vi "test_gs_v2.vi"() -> ()   [LabVIEW 2015]
uses:
  <vilib>/Native 3D Graph/xcontrol/3DPC_SurfacePlot.xctl
  <vilib>/Instr/_visa.llb/VISA Flush IO Buffer Mask.ctl
panel:
  in  "Tab Control":enum32{"Page 1", "Page 2"}(tab)
  in  "stop":bool
  out "x":string
  out "3D Graph":refnum<class "Base Datatype.lvclass">[](xcontrol)
  in  "Ramp Z to:":string(combo)
  in  "Ramp Y to:":string(combo)
  in  "Ramp X to:":string(combo)
  in  "Z-axis Persistence heater ON/OFF":bool
  in  "Y-axis Persistence heater ON/OFF":bool
  in  "Z-axis port name":refnum<visa-resource-name>
  in  "Y-axis port name":refnum<visa-resource-name>
  in  "X-axis Persistence heater ON/OFF":bool
  in  "X-axis port name":refnum<visa-resource-name>
  out "B_x":dbl
  out "B_y":dbl
  out "B_z":dbl
  in  "Field strength in Tesla":dbl min=0.0 max=9.0
  in  "beta in degrees 0 to   180":dbl min=0.0 max=180.0
  in  "alpha in degrees 0 to 360":dbl min=0.0 max=360.0
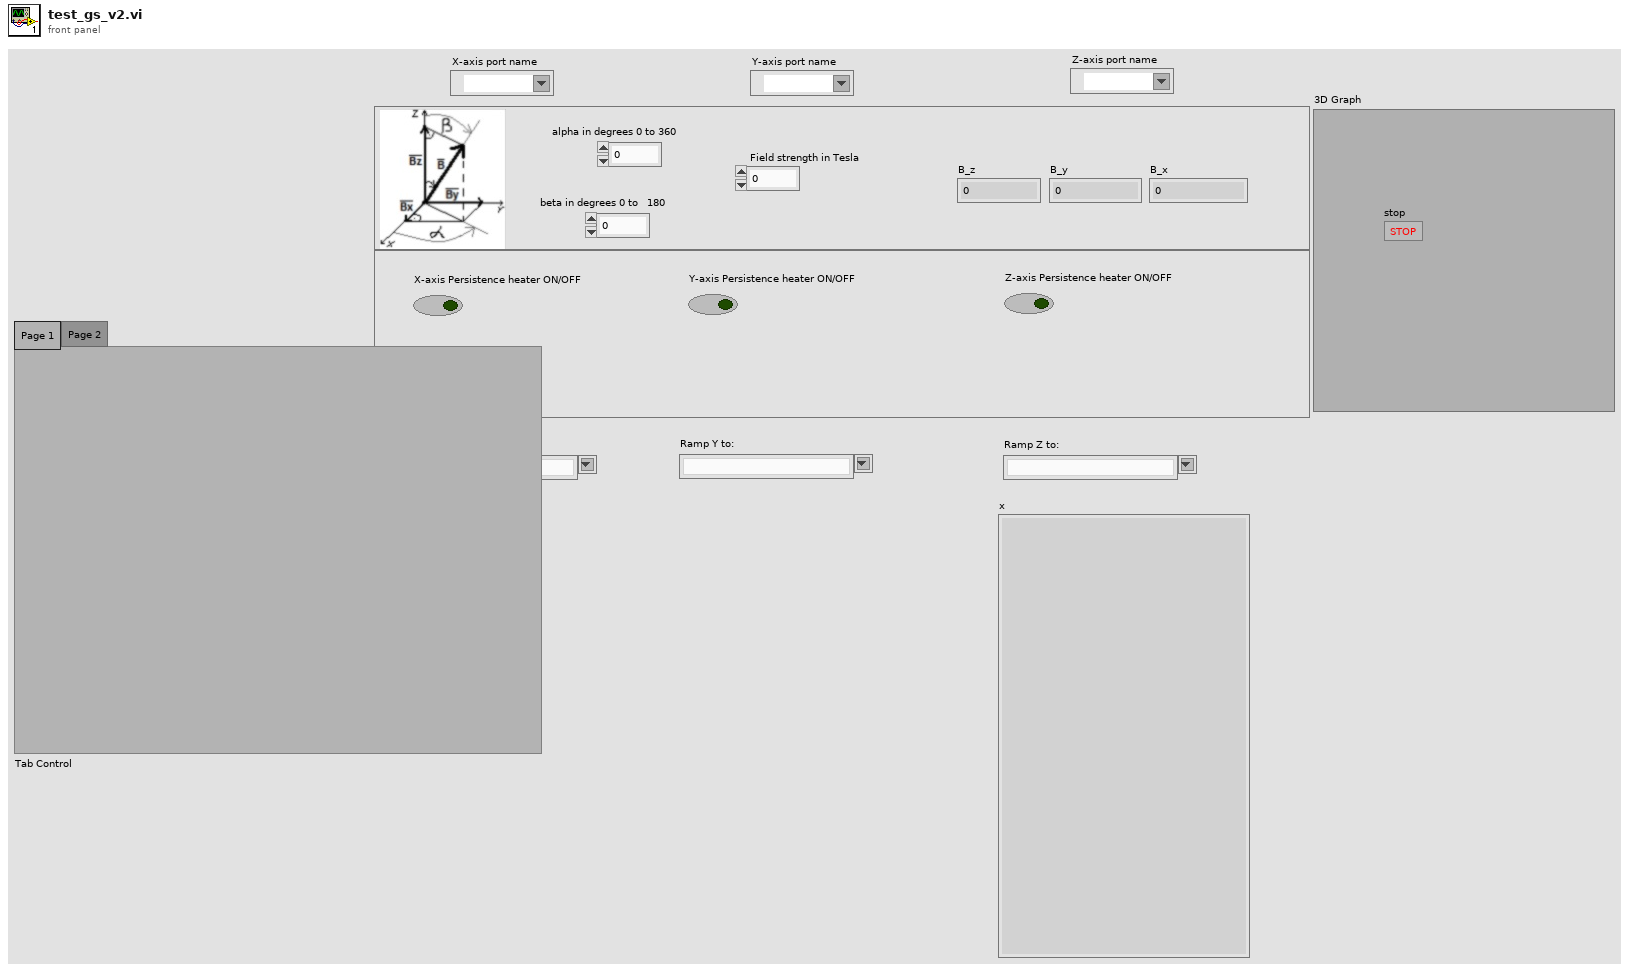
[diagram p1: front panel]
types:
  T1 = typedef "VISA Flush IO Buffer Mask.ctl" = u16
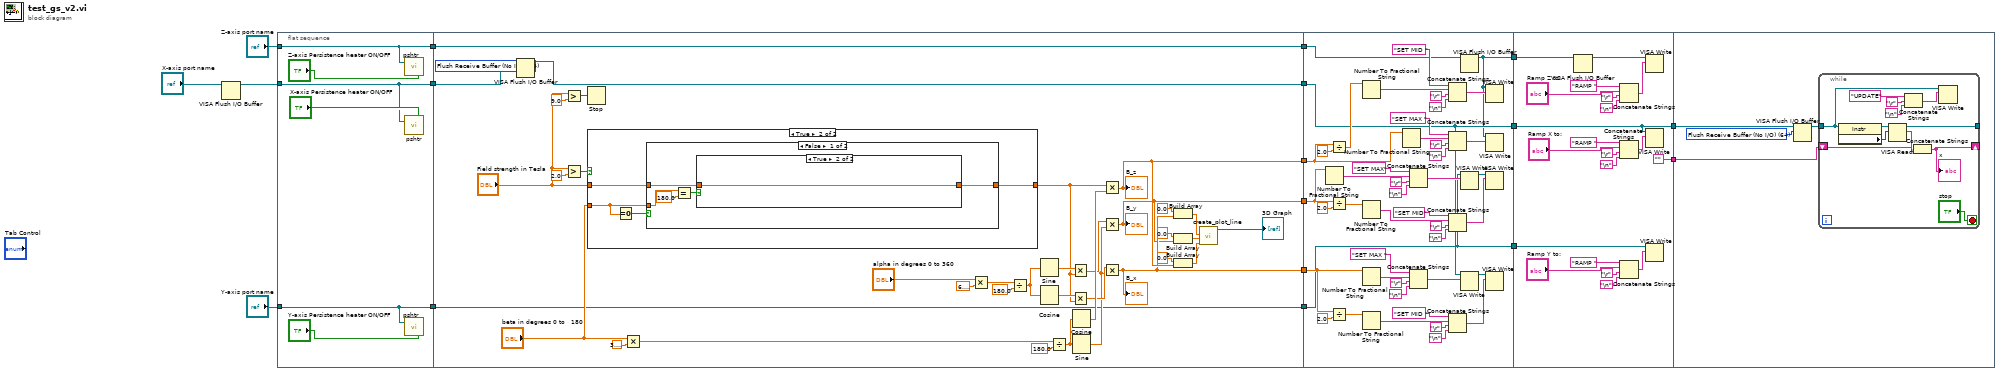
[diagram p0: block diagram]
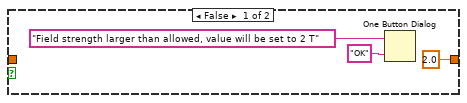
[diagram p3: hidden frame]
diagram:
  n1 = VISA Flush I/O Buffer(VISA resource name="X-axis port name") -> (VISA resource name out=w1:refnum<visa-resource-name>)  [unwired: 2 in, 1 out]
  n2 = flat-sequence {
    tunnel: "Z-axis port name" -> [w19]
    tunnel: "Y-axis port name" -> [w20]
    tunnel: w1 -> [w21]
    tunnel: [w21] -> w10
    tunnel: [w20] -> w9
    tunnel: [w19] -> w8
    tunnel: [w26] -> w16
    tunnel: [w33] -> w15
    tunnel: [w32] -> w14
    tunnel: [w31] -> w13
    tunnel: [w30] -> w12
    tunnel: [w29] -> w11
    tunnel: w10 -> [w27]
    tunnel: w9 -> [w33]
    tunnel: w8 -> [w32]
    tunnel: w16 -> [w84]
    tunnel: w15 -> [w83]
    tunnel: w14 -> [w78]
    tunnel: w13 -> [w89]
    tunnel: w12 -> [w91]
    tunnel: w11 -> [w88]
    tunnel: [w84] -> w7
    tunnel: [w83] -> w6
    tunnel: [w77] -> w5
    tunnel: w7 -> [w122]
    tunnel: w6 -> [w129]
    tunnel: w5 -> [w124]
    tunnel: [""] -> w4
    tunnel: [w122] -> w3
    tunnel: w4 -> [w145]
    tunnel: w3 -> [w144]
    frame #0 {
      n3 = call "pshtr.vi"("Boolean"="Z-axis Persistence heater ON/OFF", "VISA resource name"=w19) -> ()  [unwired: 1 in]
      n4 = call "pshtr.vi"("Boolean"="X-axis Persistence heater ON/OFF", "VISA resource name"=w21) -> ()  [unwired: 1 in]
      n5 = call "pshtr.vi"("Boolean"="Y-axis Persistence heater ON/OFF", "VISA resource name"=w20) -> ()  [unwired: 1 in]
    }
    frame #1 {
      w25 = T1 64 items=["Flush Receive Buffer"=16, "Write Transmit Buffer to Device"=32, "Flush Receive Buffer (No I/O)"=64, "Flush Transmit Buffer"=128] ("Mask")
      n6 = VISA Flush I/O Buffer(VISA resource name=w27, mask (16)=w25) -> (VISA resource name out=w26:refnum<visa-resource-name>)  [unwired: 1 in, 1 out]
      n7 = Greater?(x="Field strength in Tesla", y=9.0) -> (0:w34:bool)
      n8 = Greater?(x="Field strength in Tesla", y=2.0) -> (0:w40:bool)
      n9 = Stop(stop? (T)=w34) -> ()
      n10 = case shown="True" w40 {
        tunnel: "beta in degrees 0 to   180" -> [_ w64]
        tunnel: "Field strength in Tesla" -> [w62 w66]
        tunnel: [w62 w63] -> w37
        frame False {
        }
        frame True {
          n11 = Equal To 0?(x=w64) -> (x = 0?=w65:bool)
          n12 = case shown="False" w65 {
            tunnel: w66 -> [w67 w76]
            tunnel: w64 -> [w70 _]
            tunnel: [w68 w76] -> w63
            frame False {
              n13 = Equal?(x=w70, y=180.0) -> (x = y?=w69:bool)
              n14 = case shown="True" w69 {
                tunnel: [2.0 w75] -> w68
                tunnel: w67 -> [_ w75]
                frame False {
                  n15 = One Button Dialog(message="Field strength larger than allowed, value will be set to 2 T", button name ("OK")="OK") -> ()  [unwired: 1 out]
                }
                frame True {
                }
              }
            }
            frame True {
            }
          }
        }
      }
      n16 = Multiply(x="beta in degrees 0 to   180", y=3.141592653589793) -> (x*y=w57:dbl)
      n17 = Multiply(x="alpha in degrees 0 to 360", y=6.283185307179586) -> (x*y=w60:dbl)
      n18 = Divide(x=w60, y=180.0) -> (x/y=w53:dbl)
      n19 = Sine(x=w53) -> (sin(x)=w51:dbl)
      n20 = Cosine(x=w53) -> (cos(x)=w52:dbl)
      n21 = Divide(x=w57, y=180.0) -> (x/y=w54:dbl)
      n22 = Multiply(x=w51, y=w37) -> (x*y=w50:dbl)
      n23 = Multiply(x=w52, y=w37) -> (x*y=w49:dbl)
      n24 = Cosine(x=w54) -> (cos(x)=w55:dbl)
      n25 = Sine(x=w54) -> (sin(x)=w48:dbl)
      n26 = Multiply(x=w37, y=w55) -> (x*y=w31:dbl)
      "B_z" <- w31
      n27 = Multiply(x=w50, y=w48) -> (x*y=w29:dbl)
      "B_y" <- w29
      n28 = Multiply(x=w49, y=w48) -> (x*y=w30:dbl)
      "B_x" <- w30
      n29 = Build Array(0.0 ("element"), w30) -> (w44:dbl[])
      n30 = Build Array(0.0 ("element"), w29) -> (w46:dbl[])
      n31 = Build Array(0.0 ("element"), w31) -> (w42:dbl[])
      n32 = call <vilib>:"create_plot_line.vi"("z vector"=w42, "y vector"=w46, "x vector"=w44) -> ("plots out"=→"3D Graph":refnum<class "Base Datatype.lvclass">[])  [unwired: 2 in, 6 out]
    }
    frame #2 {
      n33 = Number To Fractional String(number=w88) -> (F-format string=w107:string)  [unwired: 3 in]
      n34 = Divide(x=w89, y=2.0) -> (x/y=w85:dbl)
      n35 = Divide(x=w88, y=2.0) -> (x/y=w86:dbl)
      n36 = Divide(x=w91, y=2.0) -> (x/y=w90:dbl)
      n37 = Number To Fractional String(number=w85) -> (F-format string=w96:string)  [unwired: 3 in]
      n38 = Number To Fractional String(number=w86) -> (F-format string=w94:string)  [unwired: 3 in]
      n39 = Number To Fractional String(number=w91) -> (F-format string=w108:string)  [unwired: 3 in]
      n40 = Number To Fractional String(number=w90) -> (F-format string=w95:string)  [unwired: 3 in]
      n41 = Number To Fractional String(number=w89) -> (F-format string=w109:string)  [unwired: 3 in]
      n42 = Concatenate Strings("SET MAX" ("string"), w107, "\r", "\n") -> (w118:string)
      n43 = Concatenate Strings("SET MAX " ("string"), w108, "\r", "\n") -> (w120:string)
      n44 = Concatenate Strings("SET MID " ("string"), w96, "\r", "\n") -> (w103:string)
      n45 = Concatenate Strings("SET MAX " ("string"), w109, "\r", "\n") -> (w116:string)
      n46 = Concatenate Strings("SET MID" ("string"), w94, "\r", "\n") -> (w82:string)
      n47 = Concatenate Strings("SET MID " ("string"), w95, "\r", "\n") -> (w79:string)
      n48 = VISA Flush I/O Buffer(VISA resource name=w78) -> (VISA resource name out=w77:refnum<visa-resource-name>)  [unwired: 2 in, 1 out]
      n49 = VISA Write(VISA resource name=w83, write buffer=w118) -> (VISA resource name out=w81:refnum<visa-resource-name>)  [unwired: 1 in, 2 out]
      n50 = VISA Write(VISA resource name=w84, write buffer=w120) -> (VISA resource name out=w80:refnum<visa-resource-name>)  [unwired: 1 in, 2 out]
      n51 = VISA Write(VISA resource name=w77, write buffer=w103) -> ()  [unwired: 1 in, 3 out]
      n52 = VISA Write(VISA resource name=w77, write buffer=w116) -> ()  [unwired: 1 in, 3 out]
      n53 = VISA Write(VISA resource name=w81, write buffer=w82) -> ()  [unwired: 1 in, 3 out]
      n54 = VISA Write(VISA resource name=w80, write buffer=w79) -> ()  [unwired: 1 in, 3 out]
    }
    frame #3 {
      n55 = VISA Flush I/O Buffer(VISA resource name=w124) -> (VISA resource name out=w123:refnum<visa-resource-name>)  [unwired: 2 in, 1 out]
      n56 = Concatenate Strings("RAMP " ("string"), "Ramp Z to:", "\r", "\n") -> (w136:string)
      n57 = Concatenate Strings("RAMP " ("string"), "Ramp X to:", "\r", "\n") -> (w140:string)
      n58 = Concatenate Strings("RAMP " ("string"), "Ramp Y to:", "\r", "\n") -> (w138:string)
      n59 = VISA Write(VISA resource name=w123, write buffer=w136) -> ()  [unwired: 1 in, 3 out]
      n60 = VISA Write(VISA resource name=w122, write buffer=w140) -> ()  [unwired: 1 in, 3 out]
      n61 = VISA Write(VISA resource name=w129, write buffer=w138) -> ()  [unwired: 1 in, 3 out]
    }
    frame #4 {
      w142 = T1 64 items=["Flush Receive Buffer"=16, "Write Transmit Buffer to Device"=32, "Flush Receive Buffer (No I/O)"=64, "Flush Transmit Buffer"=128] ("Mask")
      n62 = VISA Flush I/O Buffer(VISA resource name=w144, mask (16)=w142) -> (VISA resource name out=w143:refnum<visa-resource-name>)  [unwired: 1 in, 1 out]
      n63 = while {
        tunnel: [w157] -> _
        shift-right: [w151] -> _
        shift-left: w145 -> [w152]
        tunnel: w143 -> [w147]
        stop <- "stop" stop-if-true
        n64 = property class="Instr"(reference=w147) -> (reference out=w154:refnum<visa-resource-name>, "Serial Settings:Number of Bytes at Serial Port"=w155:u32)  [unwired: 1 in, 1 out]
        n65 = VISA Read(VISA resource name=w154, byte count=w155) -> (VISA resource name out=w157:refnum<visa-resource-name>, read buffer=w153:string)  [unwired: 1 in, 2 out]
        n66 = Concatenate Strings("UPDATE" ("write buffer"), "\r", "\n") -> (w149:string)
        n67 = Concatenate Strings(w152, w153) -> (w151:string)
        "x" <- w151
        n68 = VISA Write(VISA resource name=w147, write buffer=w149) -> ()  [unwired: 1 in, 3 out]
      }
    }
  }
